vi "CH_LM App ArbitraryMeterTrendChart.vi"(0 "Stop occurrence":refnum<k4>) -> ()   [LabVIEW 2012, in "CH_LM App.lvlib"]
uses:
  CH_LM App.lvlib
  CH_LM.lvlib
  CH_LM App DeviceListElement.ctl
  CH_LM/CH_LM Streaming Data.ctl
  CH_LM App TrendingData.ctl
panel:
  out "stopped":bool
  in  "stop2":bool
  in  "stop1":bool
  in  "OK Button":bool
  in  "List of connected meters":i32[](listbox)
  out "Live Average Chart":T1(graph)
  in  "Meter Trend Data":T2 {"Histogram"."X Values" format="%0.2f"; "Statistics"."Std. Dev." format="%#_4p"; "Statistics"."Max" format="%#_4p"; "Statistics"."Min" format="%#_4p"; "Statistics"."Mean" format="%#_4p"; "Data Cluster"."Flags" format="%.0b"; "Data Cluster"."Unit ID" format="%.0b"; "Data Cluster"."Quad Distance"."Y" format="%#.1f"; "Data Cluster"."Quad Distance"."X" format="%#.1f"; "Data Cluster"."Value" format="%#.7e"; "LabMax Device List Element"."Probe Diameter" format="%#.2g"}
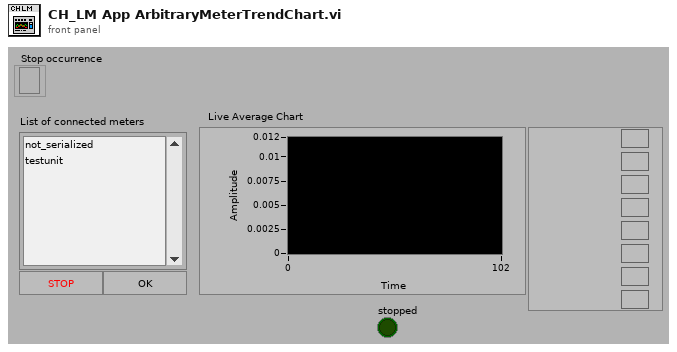
[diagram p1: front panel]
types:
  T1 = cluster{"[0]":dbl, "[1]":dbl, "[2]":dbl, "[3]":dbl, "[4]":dbl, "[5]":dbl, "[6]":dbl, "[7]":dbl}
  T2 = typedef "CH_LM App.lvlib/CH_LM App TrendingData.ctl" = cluster{"LabMax Device List Element":T3, "Data Cluster":T4, "Counts":i32, "Maximum":dbl, "Live average":dbl, "Statistics":cluster{"Mean":dbl, "Min":dbl, "Max":dbl, "Std. Dev.":dbl}, "Histogram":cluster{"H(x)":i32[], "X Values":dbl[]}, "DAQ Error":errorcluster, "stop":bool, "Quad Distance Avg.":cluster{"X":sgl, "Y":sgl}}
  T3 = typedef "CH_LM App.lvlib/CH_LM App DeviceListElement.ctl" = cluster{"Serial Number":string, "Meter Index":i32, "Probe Diameter":dbl[unit]}
  T4 = typedef "CH_LM.lvlib/CH_LM Streaming Data.ctl" = cluster{"Value":sgl, "Quad Distance":cluster{"X":sgl, "Y":sgl}, "Display Data":cluster{"Format ID":u8, "Scale ID":u8}, "Unit ID":u8, "Flags":u32, "Pulse Period":u32, "Sequence ID":u32, "Unit String":string}
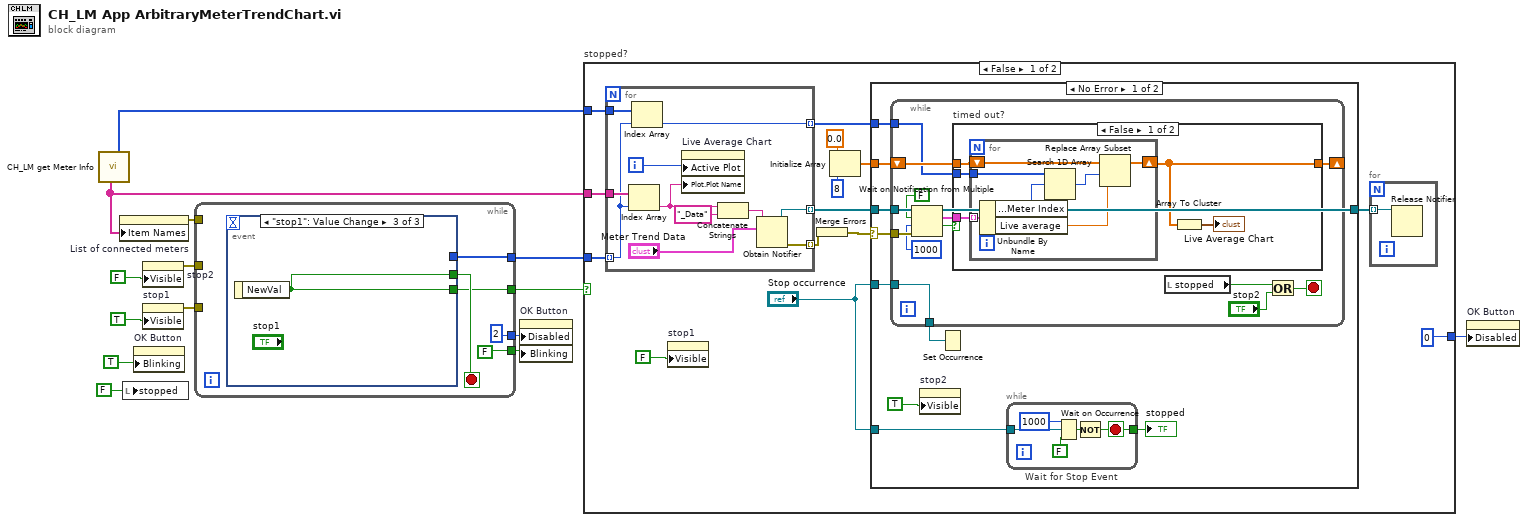
[diagram p0: block diagram]
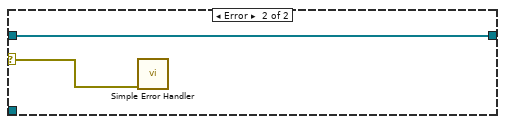
[diagram p3: hidden frame]
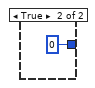
[diagram p4: hidden frame]
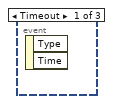
[diagram p5: hidden frame]
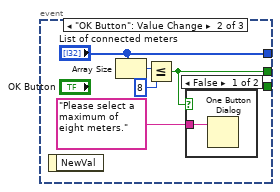
[diagram p6: hidden frame]
diagram:
  n1 = call "CH_LM get Meter Info.vi"() -> ("All Meter Indices"=w8:i32[], "All Serial Numbers"=w12:string[])  [unwired: 2 in, 8 out]
  n2 = property on="List of connected meters" class="LstBox (strict)"("Item Names"=w12) -> (error out=w14:errorcluster)  [unwired: 2 in, 1 out]
  n3 = local write "stopped"(FALSE ("stopped")) -> ()
  n4 = property on="OK Button" class="Bool"("Blinking"=TRUE) -> ()  [unwired: 2 in, 2 out]
  n5 = property on="stop2" class="Bool"("Visible"=FALSE) -> (error out=w6:errorcluster)  [unwired: 2 in, 1 out]
  n6 = property on="stop1" class="Bool"("Visible"=TRUE) -> (error out=w4:errorcluster)  [unwired: 2 in, 1 out]
  n7 = while {
    tunnel: [w18] -> w13
    tunnel: w14 -> [_]
    tunnel: [u8 2 ("Disabled")] -> w11
    tunnel: [w16] -> w10
    tunnel: w6 -> [_]
    tunnel: w4 -> [_]
    tunnel: [FALSE ("Visible")] -> w2
    stop <- w19 stop-if-true
    n8 = event shown="[2] \"stop1\": Value Change" {
      selector: _ -> [_ _ _]
      dyn-events: _ -> [_ _ _]
      timeout: _ -> [_ _ _]
      tunnel: [_ w20 w26] -> w19
      tunnel: [_ "List of connected meters" _] -> w18
      tunnel: [_ _ w26] -> w16
      event Timeout {
        n9 = event-data() -> ()  [unwired: 3 out]
      }
      event "OK Button": Value Change {
        n10 = event-data() -> ()  [unwired: 2 out]
        n11 = Array Size(array="List of connected meters") -> (size(s)=w24:i32)
        n12 = Less Or Equal?(x=w24, y=8) -> (x <= y?=w20:bool)
        n13 = case shown="False" w20 {
          tunnel: "Please select a maximum of eight meters." ("message") -> [w25 _]
          frame False {
            n14 = One Button Dialog(message=w25) -> ()  [unwired: 2 out]
          }
          frame True {
          }
        }
      }
      event "stop1": Value Change {
        n15 = event-data() -> ("NewVal"=w26:bool)  [unwired: 1 out]
      }
    }
  }
  n16 = property on="OK Button" class="Bool"("Disabled"=w11, "Blinking"=w2) -> ()  [unwired: 2 in, 2 out]
  n17 = case "stopped?" shown="False" w10 {
    tunnel: w13 -> [w40 _]
    tunnel: w12 -> [w39 _]
    tunnel: [u8 0 ("Disabled") u8 0 ("Disabled")] -> w9
    tunnel: w8 -> [w30 _]
    frame False {
      n18 = for {
        tunnel: w40 -> [w85] mode=indexing
        tunnel: w39 -> [w92]
        tunnel: [w91] -> w38 mode=indexing
        tunnel: [w90] -> w37 mode=indexing
        tunnel: w30 -> [w86]
        tunnel: [w84] -> w29 mode=indexing
        i -> [w88]
        n19 = Index Array(array=w92, index=w85) -> (element=w89:string)
        n20 = Index Array(array=w86, index=w85) -> (element=w84:i32)
        n21 = property on="Live Average Chart" class="WFChart (strict)"("Active Plot"=w88, "Plot.Plot Name"=w89) -> ()  [unwired: 2 in, 2 out]
        n22 = Concatenate Strings(w89, "_Data" ("string")) -> (w93:string)
        n23 = Obtain Notifier(name (unnamed)=w93, notification data type="Meter Trend Data") -> (notifier out=w90:refnum<notifier>, error out=w91:errorcluster)  [unwired: 2 in, 1 out]
      }
      n24 = property on="stop1" class="Bool"("Visible"=FALSE) -> ()  [unwired: 2 in, 2 out]
      n25 = Merge Errors(w38) -> (w36:errorcluster)
      n26 = Initialize Array(0.0, 8 ("dimension size")) -> (w33:dbl[])
      n27 = case shown="No Error" w36 {
        selector: w36 -> [w50 w82]
        tunnel: w37 -> [w49 w83]
        tunnel: [w49 w83] -> w35
        tunnel: w33 -> [w48 _]
        tunnel: w29 -> [w47 _]
        tunnel: "Stop occurrence" -> [w45 _]
        tunnel: "Stop occurrence" -> [w44 _]
        frame No Error {
          n28 = while {
            tunnel: w49 -> [w68]
            tunnel: w50 -> [w65]
            shift-right: [w63] -> _
            shift-left: w48 -> [w62]
            tunnel: w47 -> [w61]
            tunnel: w45 -> [w56]
            tunnel: [w56] -> w42
            stop <- w58 stop-if-true
            n29 = Wait on Notification from Multiple(0:w68, 1:FALSE ("ignore previous (F)"), 2:1000 ("timeout in ms (-1)"), 3:w65) -> (9:w64:T2[], 10:w66:bool)  [unwired: 2 out]
            n30 = case "timed out?" shown="False" w66 {
              tunnel: w64 -> [w73 _]
              tunnel: [w69 w81] -> w63
              tunnel: w62 -> [w71 w81]
              tunnel: w61 -> [w70 _]
              frame False {
                n31 = for {
                  tunnel: w73 -> [w80] mode=indexing
                  tunnel: w70 -> [w78]
                  shift-right: [w77] -> w69
                  shift-left: w71 -> [w76]
                  n32 = Unbundle By Name(w80) -> ("LabMax Device List Element.Meter Index"=w79:i32, "Live average"=w74:dbl)
                  n33 = Search 1D Array(1D array=w78, element=w79) -> (index of element=w75:i32)  [unwired: 1 out]
                  n34 = Replace Array Subset(array=w76, new element=w74, index=w75) -> (w77:dbl[])
                }
                n35 = Array To Cluster(array=w69) -> (cluster=→"Live Average Chart":T1)
              }
              frame True {
              }
            }
            n36 = local read "stopped"() -> (w57:bool)
            n37 = Or(x=w57, y="stop2") -> (x .or. y?=w58:bool)
          }
          n38 = property on="stop2" class="Bool"("Visible"=TRUE) -> ()  [unwired: 2 in, 2 out]
          n39 = Set Occurrence(w42) -> ()
          n40 = while "Wait for Stop Event" {
            tunnel: w44 -> [w54]
            tunnel: [w51] -> w43
            stop <- w51 stop-if-true
            n41 = Wait on Occurrence(1:FALSE ("ignore previous (T)"), 2:w54, 3:1000 ("ms timeout (-1)")) -> (0:w55:bool)
            n42 = Not(x=w55) -> (.not. x?=w51:bool)
          }
          "stopped" <- w43
        }
        frame Error {
          n43 = call <vilib>:"Simple Error Handler.vi"("error in (no error)"=w82) -> ()  [unwired: 1 in, 8 out]
        }
      }
      n44 = for {
        tunnel: w35 -> [w41] mode=indexing
        n45 = Release Notifier(notifier=w41) -> ()  [unwired: 1 in, 4 out]
      }
    }
    frame True {
    }
  }
  n46 = property on="OK Button" class="Bool"("Disabled"=w9) -> ()  [unwired: 2 in, 2 out]
